vi "FlattenArray.vi"(1 "Array":dbl[][](array[numeric])) -> (0 "output array":dbl[](array[numeric]))   [LabVIEW 2013]
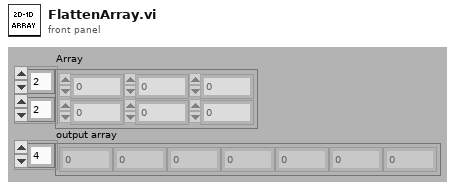
[diagram p1: front panel]
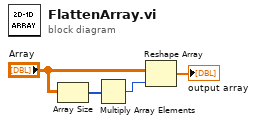
[diagram p0: block diagram]
diagram:
  n1 = Array Size(array="Array") -> (size(s)=w3:i32[])
  n2 = Multiply Array Elements(1:w3) -> (0:w2:i32)
  n3 = Reshape Array("Array", w2) -> (→"output array":dbl[])
